vi "Lockin_Vsg.vi"(8 "error in (no error)":errorcluster, 11 "Transport":refnum<class "Transport.lvclass">) -> (0 "error out":errorcluster, 3 "Transport out":refnum<class "Transport.lvclass">)   [LabVIEW 2016, in "Transport.lvclass"]
uses:
  Transport.lvclass
  Control Experiment/Typedefs/Instruments--cluster.ctl
  <userlib>/LevyLab/Krohn Hite 7008/Instrument.KH7008.lvclass
  <userlib>/LevyLab/Lockin-Multichannel/Instrument.Lockin/Instrument.Lockin.lvclass
  <userlib>/LevyLab/Levylab Instruments/Instrument Types/Cryostat/Instrument.Cryostat.lvclass
  Transport.lvclass/Transport.ctl
  Control Experiment/Control Experiment.lvclass/Control Experiment.ctl
  subVI/LockinVsg Configuration--Cluster.ctl
  Control Experiment/Control Experiment.lvclass
panel:
  in  "Tab Control":enum32{"lockin/SG Control", "Data", "Other"}(tab)
  out "elapsed time (s)":u32=76
  in  "Side Gate Channel(s)":i32[](array[numeric])=[1]
  in  "Vmax (end)":dbl=0.1 format="%#_3p"
  in  "Vmin (start)":dbl format="%#_3p"
  in  "dV":dbl=0.001 format="%#_3p"
  in  "Experiment Comments":string="describe only the experiment you're doing right now"
  in  "Experiment Folder":string="Experiment folder"
  out "T (mK)":dbl
  in  "wait after setting Vsg (ms)":u32
  in  "Initial wait (ms)":u32=1000
  in  "Physical Channel":tag="Dev2/ao0" caption="Back Gate Channel"
  in  "Sweep":enum16{"Vsg", "Vbg"}(ring)
  in  "cycles (1,2,...)":i32=1 min=1 step=1
  in  "phase":dbl
  out "Field (T)":dbl=0.5 format="%#_13g"
  in  "function (ramp)":enum16{"Ramp", "Triangle", "Sine"}(ring)
  in  "set \"Vsg\" to initial value?":bool
  out "time b/w points (ms)":u32=76
  in  "stop":bool
  out "X Lockins":cluster{dbl[], dbl[]}[](graph)
  out "X Lockins 2":cluster{dbl[], dbl[]}[](graph)
  out "G4T":cluster{dbl[], dbl[]}[](graph)
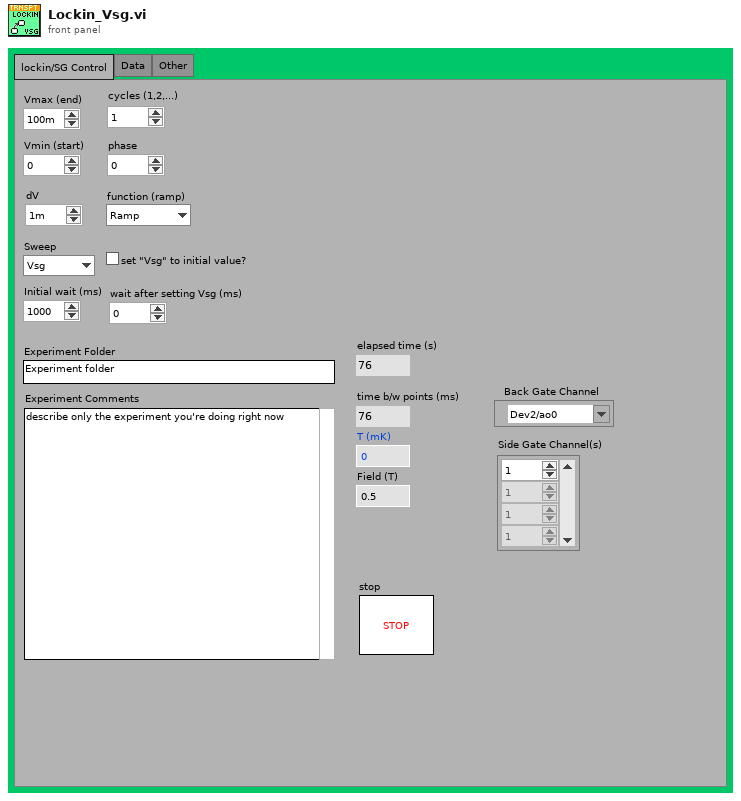
[diagram p1: front panel]
types:
  T1 = enum32{"Invalid", "Standard", "Closed", "Hidden", "Minimized", "Maximized"}
  T2 = enum32{"invalid app kind", "Development System", "Run Time System", "Student Edition", "Embedded LabVIEW", "Evaluation", "Custom"}
  T3 = typedef "Control Experiment.lvclass/Instruments--cluster.ctl" = cluster{"KH7008":refnum<class "Instrument.KH7008.lvclass">, "Lockin":refnum<class "Instrument.Lockin.lvclass">, "Temperature":refnum<class "Instrument.Cryostat.lvclass">, "Magnet":refnum<class "Instrument.Cryostat.lvclass">, "Rotator":refnum<class "Instrument.Cryostat.lvclass">, "Level":refnum<class "Instrument.Cryostat.lvclass">}
  T4 = cluster{"Core":cluster{"Current VI Reference":refnum<vi>, "Close Panel on Exit?":bool}, "Transport":refnum<class "Transport.lvclass">, "SweepControl":refnum<class "SweepControl.lvclass">, "Control Experiment":refnum<class "Control Experiment.lvclass">, "Instruments":T3, "Time":dbl, "Temperature":dbl, "Magnet":dbl, "Sweep Values":dbl[], "Results":dbl[][], "X Results":dbl[], "Y Results":dbl[], "X Results (all)":dbl[][], "Y Results (all)":dbl[][], "size":i32, "index":i32, "ms [0]":u32, "ms [i]":u32}
  T5 = cluster{"Current VI Reference":refnum<vi>, "Close Panel on Exit?":bool}
  T6 = enum32{"Bad", "Idle", "Run top level", "Running"}
  T7 = cluster{"I-":i32, "I+":i32, "V1-":i32, "V1+":i32, "V2-":i32, "V2+":i32}
  T8 = typedef "Transport.lvclass/LockinVsg Configuration--Cluster.ctl" = cluster{"Vsg Values":dbl[]}
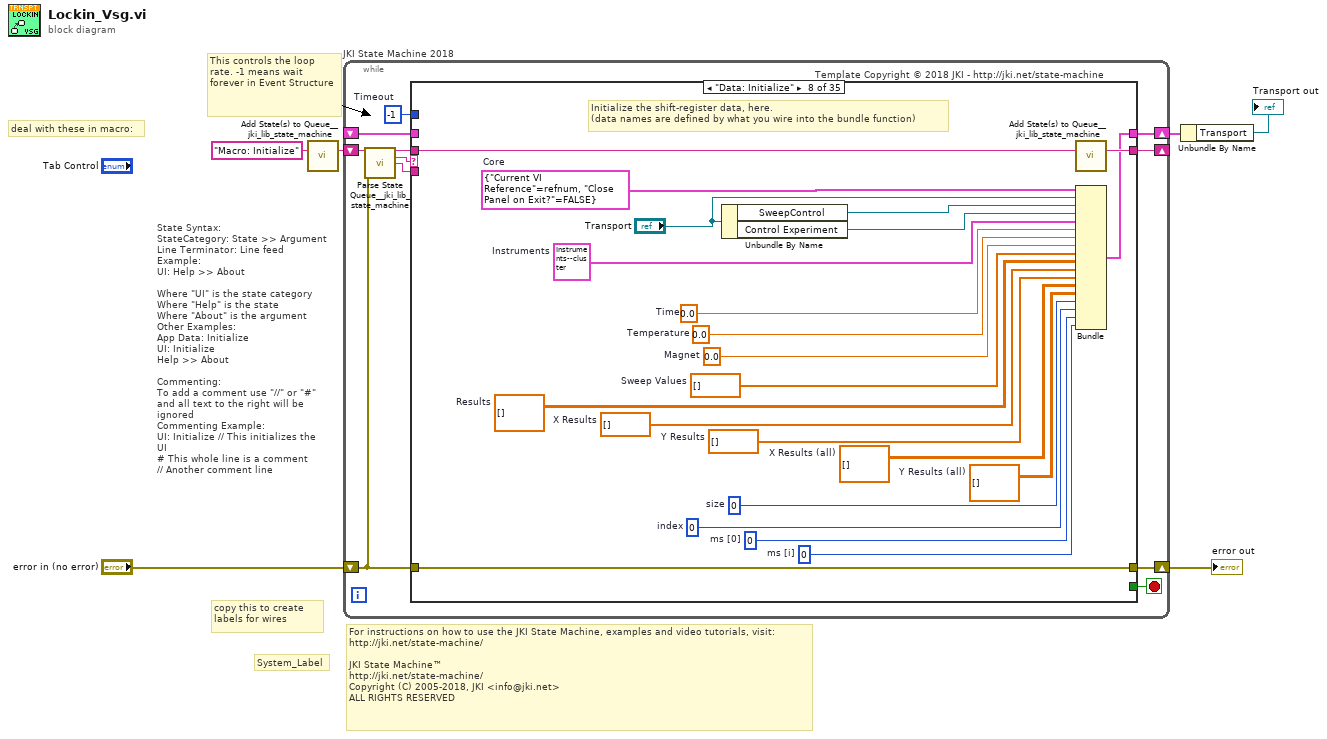
[diagram p0: block diagram]
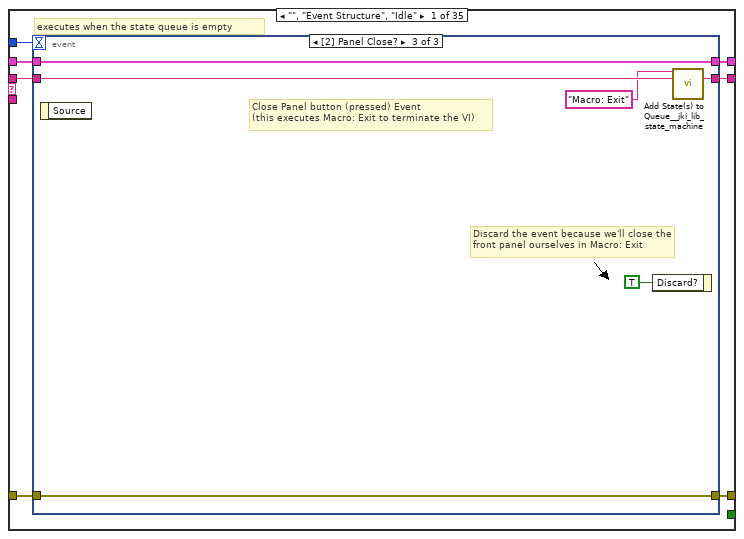
[diagram p2: hidden frame]
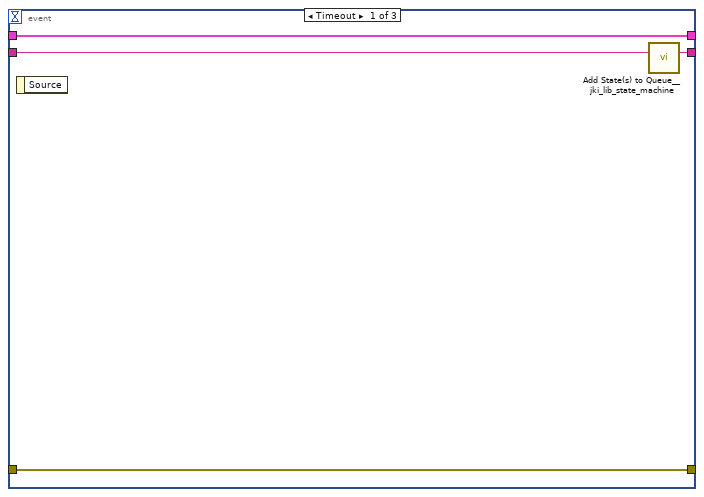
[diagram p3: hidden frame]
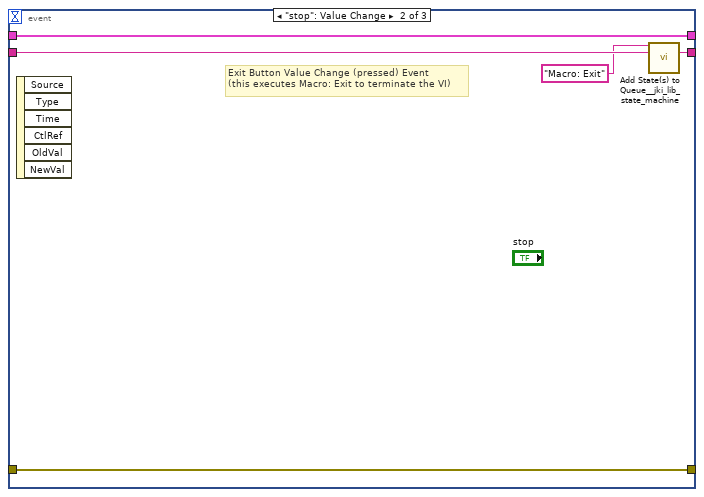
[diagram p4: hidden frame]
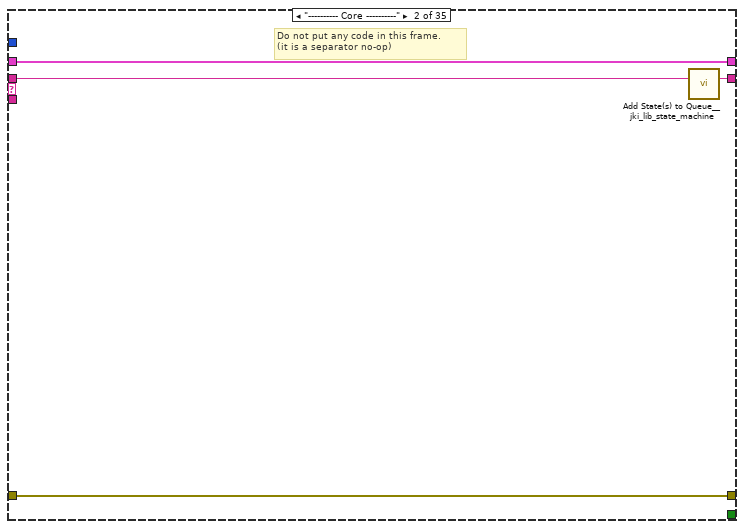
[diagram p5: hidden frame]
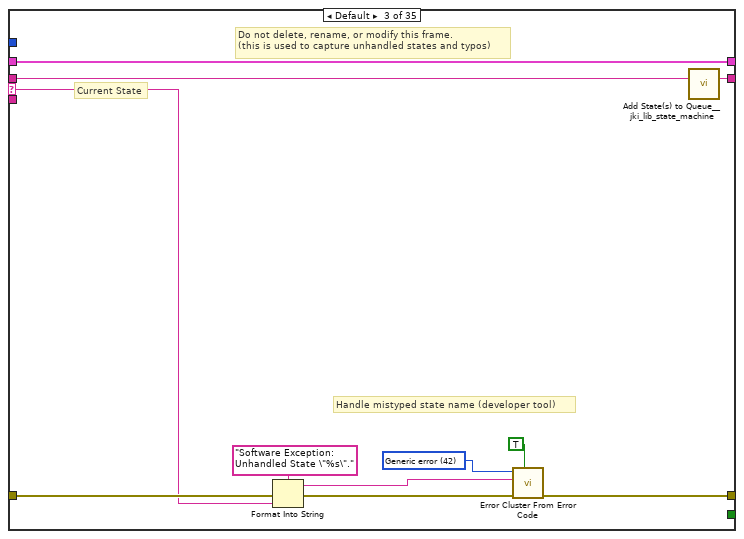
[diagram p6: hidden frame]
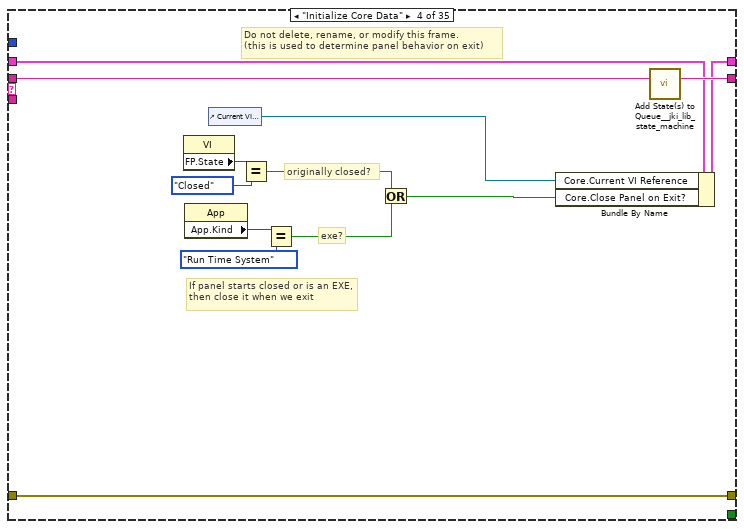
[diagram p7: hidden frame]
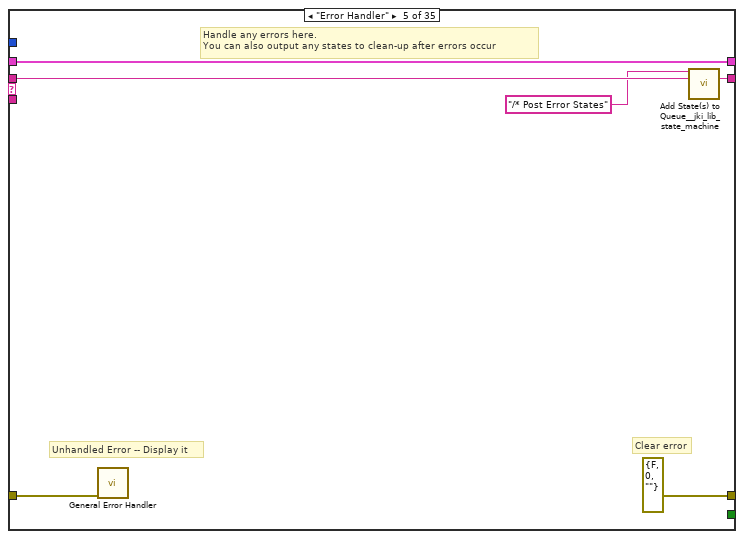
[diagram p8: hidden frame]
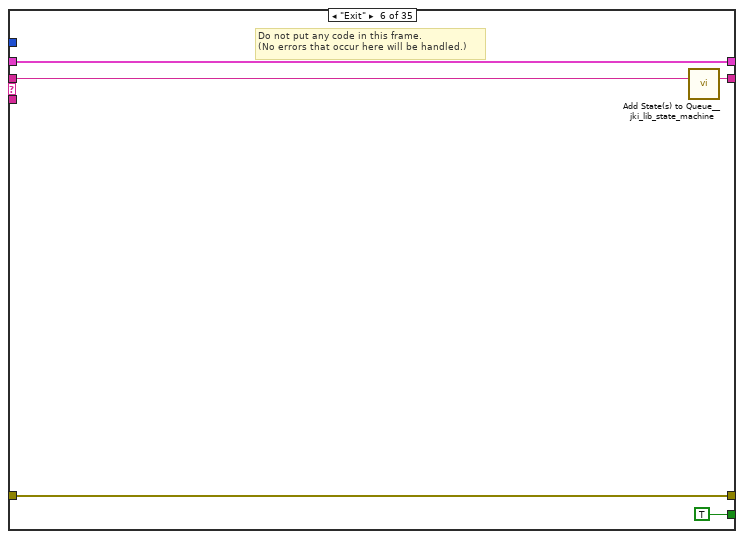
[diagram p9: hidden frame]
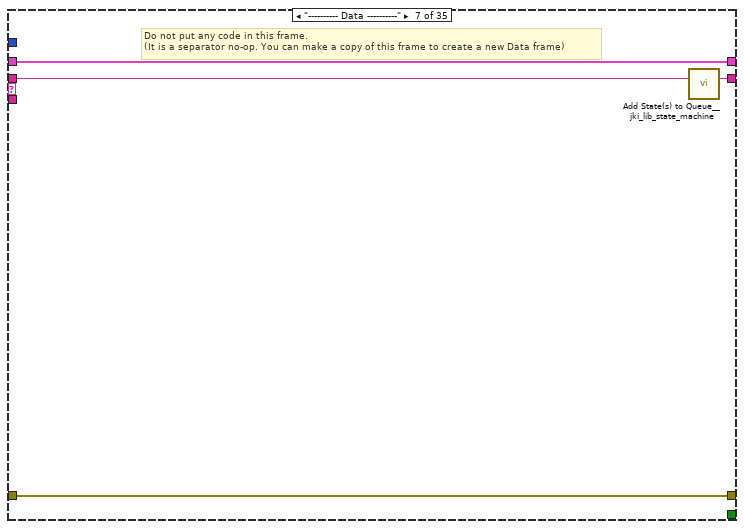
[diagram p10: hidden frame]
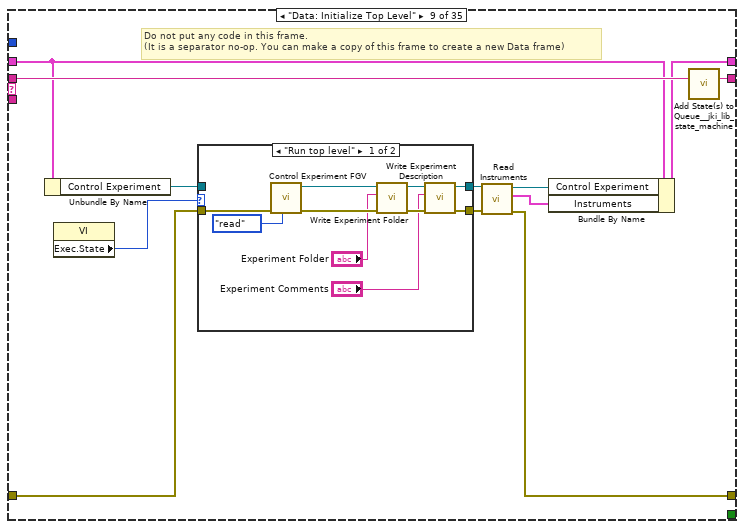
[diagram p11: hidden frame]
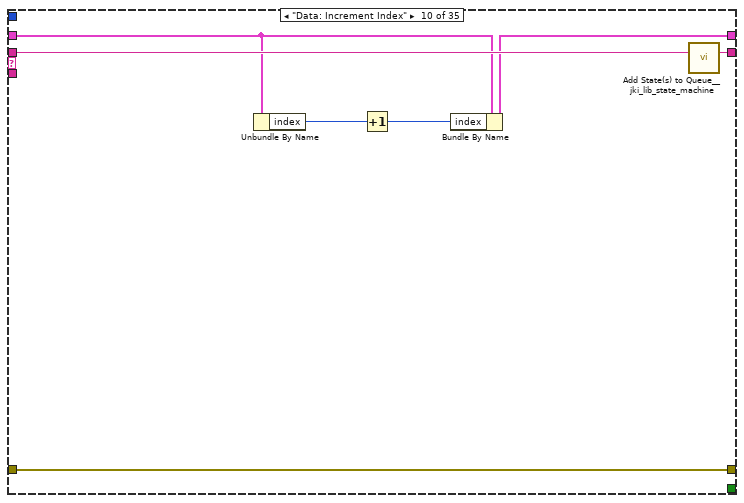
[diagram p13: hidden frame]
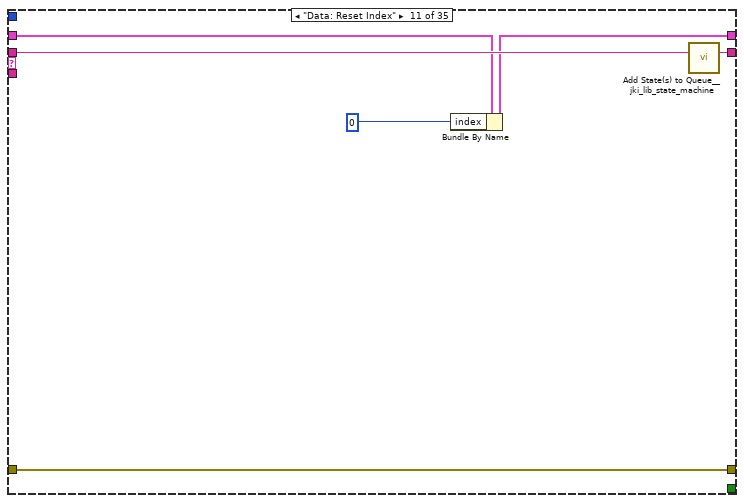
[diagram p14: hidden frame]
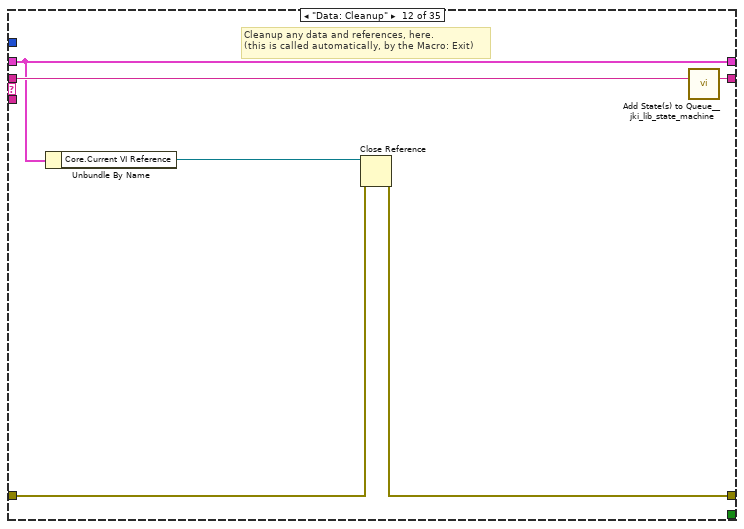
[diagram p15: hidden frame]
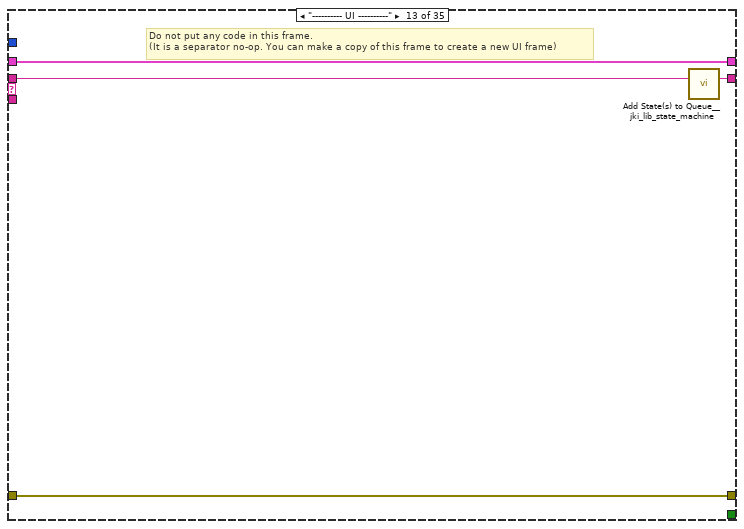
[diagram p16: hidden frame]
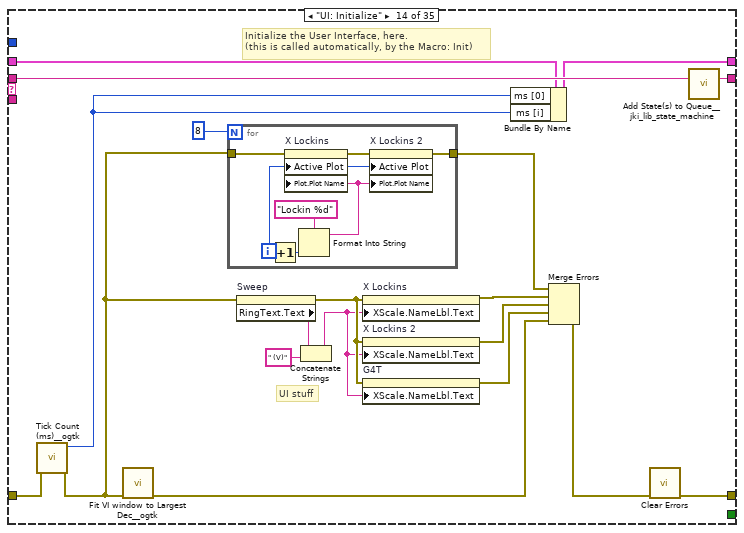
[diagram p17: hidden frame]
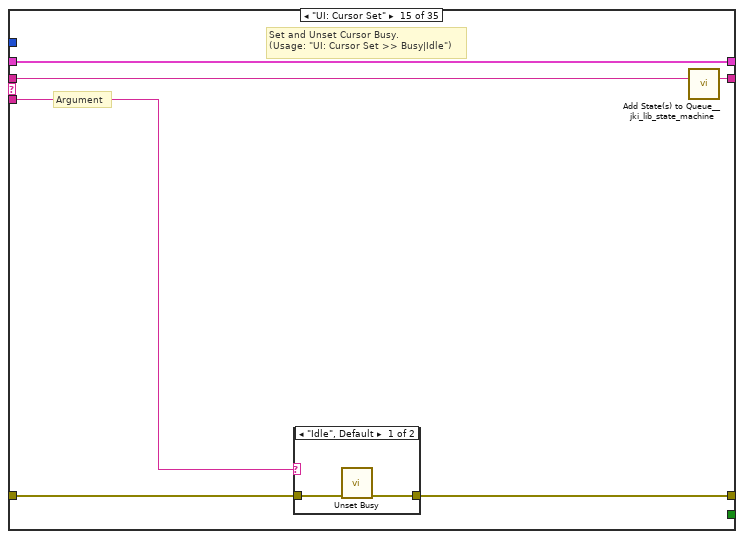
[diagram p18: hidden frame]
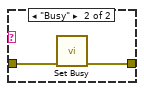
[diagram p19: hidden frame]
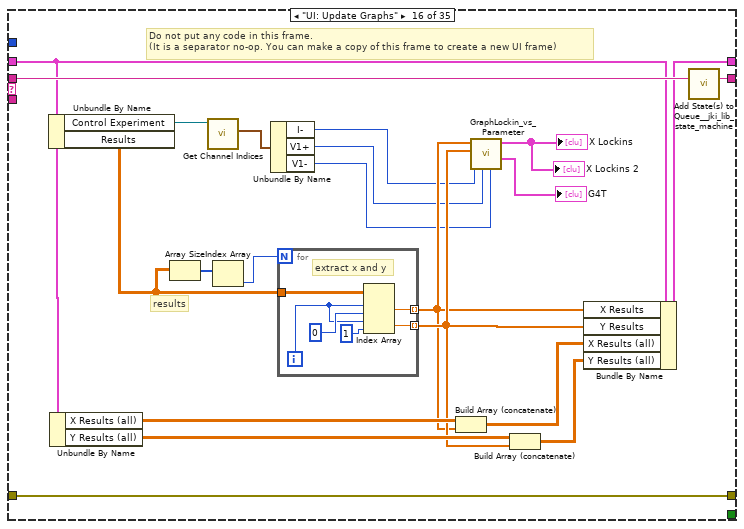
[diagram p20: hidden frame]
diagram:
  # "deal with these in macro:"
  # "For instructions on how to use the JKI State Machine, examples and video tutorials, visit:\nhttp://jki.net/state-machine/\n\nJKI State Machine™\nhttp://jki.net/state-machine/\nCopyright (C) 2005-2018, JKI <info@jki.net>\nALL RIGHTS RESERVED"
  # "State Syntax:\nStateCategory: State >> Argument\nLine Terminator: Line feed\nExample:\nUI: Help >> About\n\nWhere \"UI\" is the state category\nWhere \"Help\" is the state\nWhere \"About\" is the argument\nOther Examples:\nApp Data: Initialize\nUI: Initialize\nHelp >> About\n\nCommenting:\nTo add a comment use \"//\" or \"#\" and all text to the right will be ignored\nCommenting Example:\nUI: Initialize // This initializes the UI\n# This whole line is a comment\n// Another comment line"
  # "copy this to create labels for wires"
  # "This controls the loop rate. -1 means wait forever in Event Structure"
  # "System_Label"
  n1 = call <vilib>:"Add State(s) to Queue__jki_lib_state_machine.vi"("State(s) in (\"\")"="Macro: Initialize") -> ("States Out"=w6:string)  [unwired: 14 in]
  n2 = while "JKI State Machine 2018" {
    shift-right: [w10] -> w4
    shift-left: _ -> [w9]
    shift-right: [w13] -> w2
    shift-left: "error in (no error)" -> [w7]
    shift-right: [w12] -> _
    shift-left: w6 -> [w14]
    stop <- w11 stop-if-true
    w8 = -1  # Timeout
    # "Template Copyright © 2018 JKI - http://jki.net/state-machine"
    n3 = call <vilib>:"Parse State Queue__jki_lib_state_machine.vi"("State Queue"=w14, "Error In (no error)"=w7) -> ("Remaining States"=w16:string, "Current State"=w17:string, "Arguments"=w15:string)  [unwired: 11 in]
    n4 = case shown="\"Data: Initialize\"" w17 {
      selector: w17 -> [_ _ w44 _ _ _ _ _ _ _ _ _ _ _ _ _ _ _ _ _ _ _ _ _ _ _ _ _ _ _ _ _ _ _ _]
      tunnel: w16 -> [w24 w43 w48 w67 w73 w78 w82 w104 w116 w135 w141 w147 w151 w170 w183 w208 w227 w234 w303 w308 w326 w336 w340 w355 w359 w368 w378 w397 w408 w416 w423 w427 w431 w461 w480]
      tunnel: w15 -> [_ _ _ _ _ _ _ _ _ _ _ _ _ _ w178 _ _ w228 _ _ _ _ _ _ _ _ _ _ _ _ _ _ _ _ _]
      tunnel: w9 -> [w22 w40 w46 w60 w70 w76 w79 _ w106 w129 w138 w142 w148 w154 w181 w201 w222 w230 w300 w306 w318 w333 w337 w344 w356 w366 w376 w394 w401 w411 w419 w424 w428 w444 w476]
      tunnel: [w21 w41 w50 w64 errorcluster {"status"=FALSE, "code"=0, "source"=""} ("error out") w75 w80 w101 w107 w133 w139 w143 w149 w159 w179 w206 w215 w231 w301 w304 w324 w334 w338 w353 w357 w360 w373 w395 w402 w413 w421 w425 w429 w438 w474] -> w13
      tunnel: w7 -> [w20 w41 w49 w64 w69 w75 w80 w101 w108 w133 w139 w144 w149 w156 w180 w206 w224 w232 w301 w304 w324 w334 w338 w353 w357 w361 w374 w395 w404 w414 w421 w425 w429 w439 w475]
      tunnel: [w23 w42 w47 w66 w72 w77 w81 w103 w115 w134 w140 w146 w150 w169 w182 w207 w226 w233 w302 w307 w325 w335 w339 w354 w358 w367 w377 w396 w407 w415 w422 w426 w430 w460 w479] -> w12
      tunnel: [_ _ _ _ _ TRUE _ _ _ _ _ _ _ _ _ _ _ _ _ _ _ _ _ _ _ _ _ _ _ _ _ _ _ _ _] -> w11
      tunnel: [w19 w40 w46 w65 w70 w76 w79 w102 w105 w132 w137 w142 w148 w153 w181 w202 w221 w230 w300 w306 w318 w333 w337 w343 w356 w366 w376 w394 w400 w410 w418 w424 w428 w444 w476] -> w10
      tunnel: w8 -> [w18 _ _ _ _ _ _ _ _ _ _ _ _ _ _ _ _ _ _ _ _ _ _ _ _ _ _ _ _ _ _ _ _ _ _]
      frame "", "Event Structure", "Idle" {
        # "executes when the state queue is empty"
        n5 = event shown="[2] Panel Close?" {
          selector: _ -> [_ _ _]
          dyn-events: _ -> [_ _ _]
          timeout: w18 -> [_ _ _]
          tunnel: w24 -> [w28 w33 w39]
          tunnel: [w27 w32 w38] -> w23
          tunnel: w22 -> [w25 w30 w36]
          tunnel: [w26 w31 w37] -> w21
          tunnel: w20 -> [w26 w31 w37]
          tunnel: [w25 w30 w36] -> w19
          event Timeout {
            n6 = event-data() -> ()  [unwired: 1 in, 1 out]
            n7 = call <vilib>:"Add State(s) to Queue__jki_lib_state_machine.vi"("State(s) in (\"\")"=w28) -> ("States Out"=w27:string)  [unwired: 14 in]
          }
          event "stop": Value Change {
            # "Exit Button Value Change (pressed) Event\n(this executes Macro: Exit to terminate the VI)"
            n8 = event-data() -> ()  [unwired: 1 in, 6 out]
            n9 = call <vilib>:"Add State(s) to Queue__jki_lib_state_machine.vi"("State(s) in Front (\"\")"="Macro: Exit", "State(s) in (\"\")"=w33) -> ("States Out"=w32:string)  [unwired: 13 in]
          }
          event Panel Close? {
            # "Discard the event because we'll close the front panel ourselves in Macro: Exit"
            # "Close Panel button (pressed) Event\n(this executes Macro: Exit to terminate the VI)"
            n10 = event-data() -> ()  [unwired: 1 in, 1 out]
            n11 = event-data("Discard?"=TRUE) -> ()  [unwired: 1 in, 1 out]
            n12 = call <vilib>:"Add State(s) to Queue__jki_lib_state_machine.vi"("State(s) in Front (\"\")"="Macro: Exit", "State(s) in (\"\")"=w39) -> ("States Out"=w38:string)  [unwired: 13 in]
          }
        }
      }
      frame "---------- Core ----------" {
        # "Do not put any code in this frame.\n(it is a separator no-op)"
        n13 = call <vilib>:"Add State(s) to Queue__jki_lib_state_machine.vi"("State(s) in (\"\")"=w43) -> ("States Out"=w42:string)  [unwired: 14 in]
      }
      frame Default {
        w53 = 42 items=["No error", "Argument error", "Memory is full", "Out of zone", "End of file", "File already open", "Generic file I/O error", "File not found", "File permission error", "Disk is full", "Duplicate path", "Too many files open", "System feature not enabled", "Resource file not found", "Cannot add resource", "Resource not found", "Image not found", "Image memory error", "Pen does not exist", "Config type invalid", "Config token not found", "Config parse error", "Config memory error", "Bad external code format", "Bad external code offset", "External code not present", "Null window", "Destroy window error", "Null menu", "Print aborted", "Bad print record", "Print driver error", "Windows error during printing", "Memory error during printing", "Print dialog error", "Generic print error", "Invalid device refnum", "Device not found", "Device parameter error", "Device unit error", "Cannot open device", "Device call aborted", "Generic error", "Cancelled by user", "Object ID too low", "Object ID too high", "Object not in heap", "Unknown heap", "Unknown object (invalid DefProc)", "Unknown object (DefProc not in table)", "Message out of range", "Invalid (null) method", "Unknown message", "Manager call not supported", "Bad address", "Network operation in progress", "Network operation timed out", "Connection is busy", "Network attribute not supported", "Network error", "Address in use", "System out of memory", "Connection aborted", "Connection refused", "Not connected", "Already connected", "Connection closed", "Initialization error (interapplication manager)", "Bad occurrence", "Wait on unbound occurrence handler", "Occurrence queue overflow", "Datalog type conflict", "Unused", "Unrecognized type (interapplication manager)", "Memory corrupt", "Failed to make temporary DLL", "Old CIN version", "Drag socket not found", "Failed to load drop-object", "Failed to register OLE object", "Failed to release OLE object", "Format specifier type mismatch", "Unknown format specifier", "Too few format specifiers", "Too many format specifiers", "Scan failed", "Newer CIN version", "Error converting to variant", "Runtime menu error", "Password tampered", "Variant attribute not found", "Incompatible variant data type", "Event data is not available", "Event Store is not present", "Occurrence is not found", "Event Queue is not created", "Event info is not available", "Refnum passed is NULL", "Error retrieving Class GUID", "Error retrieving CoClass GUID", "Error retrieving TypeLib GUID.", "Bad built application magic bytes.", "Specific driver is different from the specific driver associated with the Logical Name.", "There is no session opened to the class driver.", "Max Error", "MAX - Error with config objects", "MAX - Error loading configuration", "MAX - Group not supported"]
        # "Current State"
        # "Do not delete, rename, or modify this frame.\n(this is used to capture unhandled states and typos)"
        # "Handle mistyped state name (developer tool)"
        n14 = Format Into String(format string="Software Exception: Unhandled State \"%s\"." ("message"), error in=w49, w44) -> (resulting string=w52:string, error out=w51:errorcluster)  [unwired: 1 in]
        n15 = call <vilib>:"Error Cluster From Error Code.vi"("show call chain? (False)"=TRUE, "error in (no error)"=w51, "error message (\"\")"=w52, "error code (0)"=w53) -> ("error out"=w50:errorcluster)  [unwired: 5 in]
        n16 = call <vilib>:"Add State(s) to Queue__jki_lib_state_machine.vi"("State(s) in (\"\")"=w48) -> ("States Out"=w47:string)  [unwired: 14 in]
      }
      frame "Initialize Core Data" {
        # "Do not delete, rename, or modify this frame.\n(this is used to determine panel behavior on exit)"
        # "originally closed?"
        # "exe?"
        # "If panel starts closed or is an EXE, then close it when we exit"
        n17 = property class="VI"() -> ("FP.State"=w57:T1)  [unwired: 2 in, 2 out]
        n18 = property class="App"() -> ("App.Kind"=w63:T2)  [unwired: 2 in, 2 out]
        n19 = control-ref of="Current VI Reference"() -> (w58:refnum<vi>)
        n20 = Equal?(x=w57, y=T1."Closed" ("Front Panel Window:State")) -> (x = y?=w55:bool)
        n21 = Equal?(x=w63, y=T2."Run Time System" ("Application:Kind")) -> (x = y?=w61:bool)
        n22 = Or(x=w55, y=w61) -> (x .or. y?=w59:bool)
        n23 = Bundle By Name(cluster=w60, "Core.Current VI Reference"=w58, "Core.Close Panel on Exit?"=w59) -> (w65:T4)
        n24 = call <vilib>:"Add State(s) to Queue__jki_lib_state_machine.vi"("State(s) in (\"\")"=w67) -> ("States Out"=w66:string)  [unwired: 14 in]
      }
      frame "Error Handler" {
        # "Unhandled Error -- Display it"
        # "Handle any errors here.\nYou can also output any states to clean-up after errors occur"
        # "Clear error"
        n25 = call <vilib>:"General Error Handler.vi"("error in (no error)"=w69) -> ()  [unwired: 10 in, 5 out]
        n26 = call <vilib>:"Add State(s) to Queue__jki_lib_state_machine.vi"("State(s) in Front (\"\")"="/* Post Error States", "State(s) in (\"\")"=w73) -> ("States Out"=w72:string)  [unwired: 13 in]
      }
      frame "Exit" {
        # "Do not put any code in this frame.\n(No errors that occur here will be handled.)"
        n27 = call <vilib>:"Add State(s) to Queue__jki_lib_state_machine.vi"("State(s) in (\"\")"=w78) -> ("States Out"=w77:string)  [unwired: 14 in]
      }
      frame "---------- Data ----------" {
        # "Do not put any code in this frame.\n(It is a separator no-op. You can make a copy of this frame to create a new Data frame)"
        n28 = call <vilib>:"Add State(s) to Queue__jki_lib_state_machine.vi"("State(s) in (\"\")"=w82) -> ("States Out"=w81:string)  [unwired: 14 in]
      }
      frame "Data: Initialize" {
        w85 = 0  # size
        w86 = u32 0  # ms [i]
        w87 = u32 0  # ms [0]
        w91 = 0  # index
        w92 = dbl[][] []  # Y Results (all)
        w93 = dbl[][] []  # X Results (all)
        w88 = dbl[] []  # Y Results
        w89 = dbl[] []  # X Results
        w94 = 0.0  # Time
        w95 = dbl[][] []  # Results
        w96 = dbl[] []  # Sweep Values
        w97 = 0.0  # Magnet
        w90 = 0.0  # Temperature
        w98 = T3 {"KH7008"=refnum, "Lockin"=refnum, "Temperature"=refnum, "Magnet"=refnum, "Rotator"=refnum, "Level"=refnum}  # Instruments
        w100 = T5 {"Current VI Reference"=refnum, "Close Panel on Exit?"=FALSE}  # Core
        # "Initialize the shift-register data, here.\n(data names are defined by what you wire into the bundle function)"
        n29 = Unbundle By Name("Transport") -> ("SweepControl"=w84:refnum<class "SweepControl.lvclass">, "Control Experiment"=w83:refnum<class "Control Experiment.lvclass">)
        n30 = call <vilib>:"Add State(s) to Queue__jki_lib_state_machine.vi"("State(s) in (\"\")"=w104) -> ("States Out"=w103:string)  [unwired: 14 in]
        n31 = Bundle("Core"=w100, "Transport"="Transport", "SweepControl"=w84, "Control Experiment"=w83, "Instruments"=w98, "Time"=w94, "Temperature"=w90, "Magnet"=w97, "Sweep Values"=w96, "Results"=w95, "X Results"=w89, "Y Results"=w88, "X Results (all)"=w93, "Y Results (all)"=w92, "size"=w85, "index"=w91, "ms [0]"=w87, "ms [i]"=w86) -> (w102:T4)  [unwired: 1 in]
      }
      frame "Data: Initialize Top Level" {
        # "Do not put any code in this frame.\n(It is a separator no-op. You can make a copy of this frame to create a new Data frame)"
        n32 = Unbundle By Name(w106) -> ("Control Experiment"=w109:refnum<class "Control Experiment.lvclass">)
        n33 = property class="VI"() -> ("Exec.State"=w114:T6)  [unwired: 2 in, 2 out]
        n34 = case shown="\"Run top level\"" w114 {
          tunnel: w108 -> [w126 w127]
          tunnel: [w121 w127] -> w110
          tunnel: [w120 w128] -> w111
          tunnel: w109 -> [_ w128]
          frame "Run top level" {
            n35 = call "Control Experiment FGV.vi"("Function"=enum16{"read", "write"}."read", "error in (no error)"=w126) -> ("error out"=w124:errorcluster, "Control Experiment.lvclass out"=w125:refnum<class "Control Experiment.lvclass">)  [unwired: 8 in]
            n36 = call "Write Experiment Folder.vi"("error in (no error)"=w124, "Experiment Folder"="Experiment Folder", "Control Experiment in"=w125) -> ("error out"=w122:errorcluster, "Control Experiment out"=w123:refnum<class "Control Experiment.lvclass">)  [unwired: 7 in]
            n37 = call "Write Experiment Description.vi"("error in (no error)"=w122, "Experiment Description"="Experiment Comments", "Control Experiment in"=w123) -> ("error out"=w121:errorcluster, "Control Experiment out"=w120:refnum<class "Control Experiment.lvclass">)  [unwired: 7 in]
          }
          frame "Running", Default {
          }
        }
        n38 = call "Read Instruments.vi"("error in (no error)"=w110, "Control Experiment in"=w111) -> ("error out"=w107:errorcluster, "Instruments"=w113:T3, "Control Experiment out"=w112:refnum<class "Control Experiment.lvclass">)  [unwired: 7 in]
        n39 = Bundle By Name(cluster=w106, "Control Experiment"=w112, "Instruments"=w113) -> (w105:T4)
        n40 = call <vilib>:"Add State(s) to Queue__jki_lib_state_machine.vi"("State(s) in (\"\")"=w116) -> ("States Out"=w115:string)  [unwired: 14 in]
      }
      frame "Data: Increment Index" {
        n41 = Unbundle By Name(w129) -> ("index"=w131:i32)
        n42 = Increment(x=w131) -> (x+1=w130:i32)
        n43 = Bundle By Name(cluster=w129, "index"=w130) -> (w132:T4)
        n44 = call <vilib>:"Add State(s) to Queue__jki_lib_state_machine.vi"("State(s) in (\"\")"=w135) -> ("States Out"=w134:string)  [unwired: 14 in]
      }
      frame "Data: Reset Index" {
        n45 = Bundle By Name(cluster=w138, "index"=0) -> (w137:T4)
        n46 = call <vilib>:"Add State(s) to Queue__jki_lib_state_machine.vi"("State(s) in (\"\")"=w141) -> ("States Out"=w140:string)  [unwired: 14 in]
      }
      frame "Data: Cleanup" {
        # "Cleanup any data and references, here.\n(this is called automatically, by the Macro: Exit)"
        n47 = Unbundle By Name(w142) -> ("Core.Current VI Reference"=w145:refnum<vi>)
        n48 = Close Reference(reference=w145, error in (no error)=w144) -> (error out=w143:errorcluster)
        n49 = call <vilib>:"Add State(s) to Queue__jki_lib_state_machine.vi"("State(s) in (\"\")"=w147) -> ("States Out"=w146:string)  [unwired: 14 in]
      }
      frame "---------- UI ----------" {
        # "Do not put any code in this frame.\n(It is a separator no-op. You can make a copy of this frame to create a new UI frame)"
        n50 = call <vilib>:"Add State(s) to Queue__jki_lib_state_machine.vi"("State(s) in (\"\")"=w151) -> ("States Out"=w150:string)  [unwired: 14 in]
      }
      frame "UI: Initialize" {
        # "UI stuff"
        # "Initialize the User Interface, here.\n(this is called automatically, by the Macro: Init)"
        n51 = call <userlib>:"Tick Count (ms)__ogtk.vi"("error in (no error)"=w156) -> ("error out"=w155:errorcluster, "millisecond timer value"=w152:u32)  [unwired: 9 in]
        n52 = call <userlib>:"Fit VI window to Largest Dec__ogtk.vi"("error in (no error)"=w155) -> ("error out"=w158:errorcluster)  [unwired: 5 in, 1 out]
        n53 = for {
          N: 8 -> [_]
          tunnel: [w171] -> w165
          tunnel: w155 -> [w176]
          i -> [w174]
          n54 = Increment(x=w174) -> (x+1=w172:i32)
          n55 = Format Into String(format string="Lockin %d", w172) -> (resulting string=w175:string)  [unwired: 2 in, 1 out]
          n56 = property on="X Lockins" class="XYGraph (strict)"(error in=w176, "Active Plot"=w174, "Plot.Plot Name"=w175) -> (error out=w173:errorcluster)  [unwired: 1 in, 1 out]
          n57 = property on="X Lockins 2" class="XYGraph (strict)"(error in=w173, "Active Plot"=w174, "Plot.Plot Name"=w175) -> (error out=w171:errorcluster)  [unwired: 1 in, 1 out]
        }
        n58 = property on="Sweep" class="Enum (strict)"(error in=w155) -> (error out=w164:errorcluster, "RingText.Text"=w162:string)  [unwired: 1 in, 1 out]
        n59 = Concatenate Strings(w162, " (V)" ("string")) -> (w163:string)
        n60 = property on="X Lockins" class="XYGraph (strict)"(error in=w164, "XScale.NameLbl.Text"=w163) -> (error out=w166:errorcluster)  [unwired: 1 in, 1 out]
        n61 = property on="X Lockins 2" class="XYGraph (strict)"(error in=w164, "XScale.NameLbl.Text"=w163) -> (error out=w167:errorcluster)  [unwired: 1 in, 1 out]
        n62 = property on="G4T" class="XYGraph (strict)"(error in=w164, "XScale.NameLbl.Text"=w163) -> (error out=w168:errorcluster)  [unwired: 1 in, 1 out]
        n63 = Bundle By Name(cluster=w154, "ms [0]"=w152, "ms [i]"=w152) -> (w153:T4)
        n64 = Merge Errors(w165, w166, w167, w168, w158) -> (w157:errorcluster)
        n65 = call <vilib>:"Clear Errors.vi"("error in (no error)"=w157) -> ("error out"=w159:errorcluster)  [unwired: 5 in, 1 out]
        n66 = call <vilib>:"Add State(s) to Queue__jki_lib_state_machine.vi"("State(s) in (\"\")"=w170) -> ("States Out"=w169:string)  [unwired: 14 in]
      }
      frame "UI: Cursor Set" {
        # "Argument"
        # "Set and Unset Cursor Busy.\n(Usage: \"UI: Cursor Set >> Busy|Idle\")"
        n67 = case shown="\"Idle\", Default" w178 {
          tunnel: w180 -> [w185 w187]
          tunnel: [w184 w186] -> w179
          frame "Idle", Default {
            n68 = call <vilib>:"Unset Busy.vi"("error in (no error)"=w185) -> ("error out"=w184:errorcluster)  [unwired: 10 in]
          }
          frame "Busy" {
            n69 = call <vilib>:"Set Busy.vi"("error in (no error)"=w187) -> ("error out"=w186:errorcluster)  [unwired: 9 in, 1 out]
          }
        }
        n70 = call <vilib>:"Add State(s) to Queue__jki_lib_state_machine.vi"("State(s) in (\"\")"=w183) -> ("States Out"=w182:string)  [unwired: 14 in]
      }
      frame "UI: Update Graphs" {
        # "results"
        # "Do not put any code in this frame.\n(It is a separator no-op. You can make a copy of this frame to create a new UI frame)"
        n71 = Unbundle By Name(w201) -> ("Control Experiment"=w192:refnum<class "Control Experiment.lvclass">, "Results"=w197:dbl[][])
        n72 = Unbundle By Name(w201) -> ("X Results (all)"=w200:dbl[][], "Y Results (all)"=w196:dbl[][])
        n73 = Array Size(array=w197) -> (size(s)=w204:i32[])
        n74 = call "Get Channel Indices.vi"("Control Experiment in"=w192) -> ("Indices"=w191:T7)  [unwired: 8 in, 2 out]
        n75 = Index Array(array=w204) -> (element=w203:i32)  [unwired: 1 in]
        n76 = Unbundle By Name(w191) -> ("I-"=w188:i32, "V1+"=w190:i32, "V1-"=w189:i32)
        n77 = for {
          N: w203 -> [_]
          tunnel: w197 -> [w212]
          tunnel: [w211] -> w194 mode=indexing
          tunnel: [w210] -> w195 mode=indexing
          i -> [w209]
          # "extract x and y"
          n78 = Index Array(array=w212, index (row) #1=w209, index (col) #1=0 ("disabled index (col)"), index (row) #2=w209, index (col) #2=1 ("disabled index (col)")) -> (element #1=w211:dbl, element #2=w210:dbl)
        }
        n79 = Build Array (concatenate)(w200, w194) -> (w199:dbl[][])
        n80 = call "GraphLockin_vs_Parameter.vi"("V-"=w189, "V+"=w190, "Current"=w188, "Y[ ]"=w195, "X[ ]"=w194) -> ("G(e2/h) vs Parameter"=→"G4T":cluster{"Y":dbl[], "Y":dbl[]}[], "X vs Parameter"=→"X Lockins" →"X Lockins 2":cluster{dbl[], dbl[]}[])  [unwired: 3 in, 2 out]
        n81 = Build Array (concatenate)(w196, w195) -> (w198:dbl[][])
        n82 = Bundle By Name(cluster=w201, "X Results"=w194, "Y Results"=w195, "X Results (all)"=w199, "Y Results (all)"=w198) -> (w202:T4)
        n83 = call <vilib>:"Add State(s) to Queue__jki_lib_state_machine.vi"("State(s) in (\"\")"=w208) -> ("States Out"=w207:string)  [unwired: 14 in]
      }
      frame "UI: Update Timer" {
        n84 = Unbundle By Name(w222) -> ("ms [0]"=w223:u32)
        n85 = call <userlib>:"Tick Count (ms)__ogtk.vi"("error in (no error)"=w224) -> ("error out"=w216:errorcluster, "millisecond timer value"=w220:u32)  [unwired: 9 in]
        n86 = Subtract(x=w220, y=w223) -> (x-y=w218:u32)
        n87 = call <userlib>:"MGI Milliseconds Since Last Call.vi"("Error In"=w216) -> ("ms"=→"time b/w points (ms)":u32, "Error Out"=w215:errorcluster)  [unwired: 5 in]
        n88 = Multiply(x=w218, y=u32 1000 ("x")) -> (x*y=→"elapsed time (s)":u32)
        n89 = Bundle By Name(cluster=w222, "ms [i]"=w220) -> (w221:T4)
        n90 = call <vilib>:"Add State(s) to Queue__jki_lib_state_machine.vi"("State(s) in (\"\")"=w227) -> ("States Out"=w226:string)  [unwired: 14 in]
      }
      frame "UI: Front Panel State" {
        # "Argument"
        # "Set Front Panel Open or Closed\n(Usage: \"UI: Front Panel State >> Open|Close\")"
        n91 = Unbundle By Name(w230) -> ("Core.Current VI Reference"=w229:refnum<vi>)
        n92 = case shown="\"Minimize\", \"Minimized\"" w228 {
          tunnel: w232 -> [w240 w255 w266 w279 w292]
          tunnel: [w242 w256 w268 w281 w294] -> w231
          tunnel: w229 -> [w241 w253 w267 w280 w293]
          frame "Open", "Standard", Default {
            w235 = T1."Standard" ("State")
            n93 = property class="VI"(reference=w241, error in=w240) -> (reference out=w238:refnum<vi>, error out=w239:errorcluster, "FP.State"=w237:T1)
            n94 = Not Equal?(x=w237, y=w235) -> (x != y?=w236:bool)
            n95 = case shown="True" w236 {
              tunnel: [w246 w248] -> w242
              tunnel: w239 -> [w245 w248]
              tunnel: w238 -> [w244 _]
              tunnel: w235 -> [w243 _]
              frame True {
                n96 = invoke class="VI" method="FP.Open"(reference=w244, error in=w245, "Activate"=TRUE, "State"=w243) -> (error out=w246:errorcluster)  [unwired: 1 in, 4 out]
              }
              frame False {
              }
            }
          }
          frame "Close", "Closed" {
            n97 = property class="VI"(reference=w253, error in=w255) -> (reference out=w252:refnum<vi>, error out=w254:errorcluster, "FP.State"=w250:T1)
            n98 = Not Equal?(x=w250, y=T1."Closed" ("Front Panel Window:State")) -> (x != y?=w249:bool)
            n99 = case shown="True" w249 {
              tunnel: [w257 w260] -> w256
              tunnel: w254 -> [w257 w259]
              tunnel: w252 -> [_ w258]
              frame False {
              }
              frame True {
                n100 = invoke class="VI" method="FP.Close"(reference=w258, error in=w259) -> (error out=w260:errorcluster)  [unwired: 1 in, 2 out]
              }
            }
          }
          frame "Hidden", "Hide" {
            w261 = T1."Hidden" ("State")
            n101 = property class="VI"(reference=w267, error in=w266) -> (reference out=w264:refnum<vi>, error out=w265:errorcluster, "FP.State"=w263:T1)
            n102 = Not Equal?(x=w263, y=w261) -> (x != y?=w262:bool)
            n103 = case shown="True" w262 {
              tunnel: [w272 w273] -> w268
              tunnel: w265 -> [w271 w273]
              tunnel: w264 -> [w270 _]
              tunnel: w261 -> [w269 _]
              frame True {
                n104 = invoke class="VI" method="FP.Open"(reference=w270, error in=w271, "State"=w269) -> (error out=w272:errorcluster)  [unwired: 2 in, 4 out]
              }
              frame False {
              }
            }
          }
          frame "Minimize", "Minimized" {
            w274 = T1."Minimized" ("State")
            n105 = property class="VI"(reference=w280, error in=w279) -> (reference out=w277:refnum<vi>, error out=w278:errorcluster, "FP.State"=w276:T1)
            n106 = Not Equal?(x=w276, y=w274) -> (x != y?=w275:bool)
            n107 = case shown="True" w275 {
              tunnel: [w285 w286] -> w281
              tunnel: w278 -> [w284 w286]
              tunnel: w277 -> [w283 _]
              tunnel: w274 -> [w282 _]
              frame True {
                n108 = invoke class="VI" method="FP.Open"(reference=w283, error in=w284, "State"=w282) -> (error out=w285:errorcluster)  [unwired: 2 in, 4 out]
              }
              frame False {
              }
            }
          }
          frame "Maximize", "Maximized" {
            w287 = T1."Maximized" ("State")
            n109 = property class="VI"(reference=w293, error in=w292) -> (reference out=w290:refnum<vi>, error out=w291:errorcluster, "FP.State"=w289:T1)
            n110 = Not Equal?(x=w289, y=w287) -> (x != y?=w288:bool)
            n111 = case shown="True" w288 {
              tunnel: [w298 w299] -> w294
              tunnel: w291 -> [w297 w299]
              tunnel: w290 -> [w296 _]
              tunnel: w287 -> [w295 _]
              frame True {
                n112 = invoke class="VI" method="FP.Open"(reference=w296, error in=w297, "State"=w295) -> (error out=w298:errorcluster)  [unwired: 2 in, 4 out]
              }
              frame False {
              }
            }
          }
        }
        n113 = call <vilib>:"Add State(s) to Queue__jki_lib_state_machine.vi"("State(s) in (\"\")"=w234) -> ("States Out"=w233:string)  [unwired: 14 in]
      }
      frame "---------- Macro ----------" {
        # "Do not put any code in this frame.\n(It is a separator no-op. You can make a copy of this frame to create a new Macro frame)"
        n114 = call <vilib>:"Add State(s) to Queue__jki_lib_state_machine.vi"("State(s) in (\"\")"=w303) -> ("States Out"=w302:string)  [unwired: 14 in]
      }
      frame "Macro: Initialize" {
        # "Initialization Macro\n(This is called once, when the VI starts)"
        n115 = call <vilib>:"Add State(s) to Queue__jki_lib_state_machine.vi"("State(s) in Front (\"\")"="Data: Initialize\nInitialize Core Data\nUI: Initialize\nUI: Front Panel State >> Open\nData: Initialize Top Level\nData: Reset Index\nSweep: Initialize\nMacro: Sweep", "State(s) in (\"\")"=w308) -> ("States Out"=w307:string)  [unwired: 13 in]
      }
      frame "Macro: Sweep" {
        # "Do not put any code in this frame.\n(It is a separator no-op. You can make a copy of this frame to create a new Macro frame)"
        n116 = Unbundle By Name(w318) -> ("size"=w319:i32, "index"=w323:i32)
        n117 = Decrement(x=w319) -> (x-1=w311:i32)
        n118 = Not Equal?(x=w311, y=w323) -> (x != y?=w322:bool)
        n119 = Select(t="Data: Reset Index\nConfigure: Set" ("State(s) in Front (\"\")"), s="set \"Vsg\" to initial value?", f="" ("State(s) in Front (\"\")")) -> (s? t:f=w314:string)
        n120 = call <vilib>:"Add State(s) to Queue__jki_lib_state_machine.vi"("State(s) in Front (\"\")"="File: Save\nMacro: Exit" ("State(s) in Front (\"\")"), "State(s) at Back (\"\")"=w314) -> ("States Out"=w312:string)  [unwired: 13 in]
        n121 = Select(t="Macro: Sweep" ("State(s) in Front (\"\")"), s=w322, f=w312) -> (s? t:f=w321:string)
        n122 = call <vilib>:"Add State(s) to Queue__jki_lib_state_machine.vi"("State(s) in Front (\"\")"="Configure: Set\nConfigure: Wait\nMeasure: Lockin\nMeasure: Time\nMeasure: Cryostat\nUI: Update Graphs\nUI: Update Timer\nData: Increment Index" ("State(s) in Front (\"\")"), "State(s) at Back (\"\")"=w321) -> ("States Out"=w310:string)  [unwired: 13 in]
        n123 = call <vilib>:"Add State(s) to Queue__jki_lib_state_machine.vi"("State(s) in (\"\")"=w326, "State(s) at Back (\"\")"=w310) -> ("States Out"=w325:string)  [unwired: 13 in]
      }
      frame "Macro: Exit" {
        # "Exit Macro\n(This is called once, when the VI exits)"
        n124 = Unbundle By Name(w333) -> ("Core.Close Panel on Exit?"=w332:bool)
        n125 = Select(t="UI: Front Panel State >> Close", s=w332, f="") -> (s? t:f=w329:string)
        n126 = call <vilib>:"Add State(s) to Queue__jki_lib_state_machine.vi"("State(s) in (\"\")"=w329, "State(s) at Back (\"\")"="Data: Cleanup\nExit") -> ("States Out"=w327:string)  [unwired: 13 in]
        n127 = call <vilib>:"Add State(s) to Queue__jki_lib_state_machine.vi"("State(s) in Front (\"\")"=w327, "State(s) in (\"\")"=w336) -> ("States Out"=w335:string)  [unwired: 13 in]
      }
      frame "---------- Sweep ----------" {
        # "Do not put any code in this frame.\n(It is a separator no-op. You can make a copy of this frame to create a new Macro frame)"
        n128 = call <vilib>:"Add State(s) to Queue__jki_lib_state_machine.vi"("State(s) in (\"\")"=w340) -> ("States Out"=w339:string)  [unwired: 14 in]
      }
      frame "Sweep: Initialize" {
        # "define sweep"
        # "Do not put any code in this frame.\n(It is a separator no-op. You can make a copy of this frame to create a new Macro frame)"
        n129 = call <userlib>:"Max_Min_conversion.vi"("Min"="Vmin (start)", "Max"="Vmax (end)") -> ("offset"=w346:dbl, "Amplitude"=w345:dbl)  [unwired: 8 in]
        n130 = call <userlib>:"Ramp.vi"("phase"="phase", "function (ramp)"="function (ramp)", "cycles (1,2,...)"="cycles (1,2,...)", "step size"="dV", "offset"=w346, "amplitude"=w345) -> ("Waveform Graph"=w342:dbl[])  [unwired: 3 in, 2 out]
        n131 = Array Size(array=w342) -> (size(s)=w341:i32)
        n132 = Bundle By Name(cluster=w344, "Sweep Values"=w342, "size"=w341) -> (w343:T4)
        n133 = call <vilib>:"Add State(s) to Queue__jki_lib_state_machine.vi"("State(s) in (\"\")"=w355) -> ("States Out"=w354:string)  [unwired: 14 in]
      }
      frame "---------- Configure ----------" {
        # "Do not put any code in this frame.\n(It is a separator no-op. You can make a copy of this frame to create a new Macro frame)"
        n134 = call <vilib>:"Add State(s) to Queue__jki_lib_state_machine.vi"("State(s) in (\"\")"=w359) -> ("States Out"=w358:string)  [unwired: 14 in]
      }
      frame "Configure: Wait" {
        # "Do not put any code in this frame.\n(It is a separator no-op. You can make a copy of this frame to create a new Macro frame)"
        n135 = First Call?() -> (First Call?: T/F=w362:bool)
        n136 = Select(t="Initial wait (ms)", s=w362, f="wait after setting Vsg (ms)") -> (s? t:f=w365:u32)
        n137 = call <userlib>:"Wait (ms)__ogtk.vi"("error in (no error)"=w361, "milliseconds to wait"=w365) -> ("error out"=w360:errorcluster)  [unwired: 8 in, 1 out]
        n138 = call <vilib>:"Add State(s) to Queue__jki_lib_state_machine.vi"("State(s) in (\"\")"=w368) -> ("States Out"=w367:string)  [unwired: 14 in]
      }
      frame "Configure: Set" {
        # "Do not put any code in this frame.\n(It is a separator no-op. You can make a copy of this frame to create a new Macro frame)"
        n139 = Unbundle By Name(w376) -> ("Instruments.Lockin"=w375:refnum<class "Instrument.Lockin.lvclass">, "Sweep Values"=w372:dbl[], "index"=w371:i32)
        n140 = Index Array(array=w372, index=w371) -> (element=w370:dbl)
        n141 = case shown="\"Vsg\", Default" "Sweep" {
          tunnel: w375 -> [w383 _]
          tunnel: w374 -> [w381 w392]
          tunnel: [w380 w390] -> w373
          tunnel: w370 -> [w379 w391]
          frame "Vsg", Default {
            n142 = for {
              tunnel: "Side Gate Channel(s)" -> [w388] mode=indexing
              tunnel: w379 -> [w387]
              tunnel: w383 -> [w389]
              tunnel: [w384] -> _
              tunnel: w381 -> [w386]
              tunnel: [w385] -> w380
              n143 = call <userlib>:"configAO_DC.vi"("error in (no error)"=w386, "DC (V)"=w387, "AO Channel"=w388, "Instrument.Lockin in"=w389) -> ("error out"=w385:errorcluster, "Instrument.Lockin out"=w384:refnum<class "Instrument.Lockin.lvclass">)  [unwired: 6 in]
            }
          }
          frame "Vbg" {
            n144 = call <vilib>:"Voltage Update.vi"("error in (no error)"=w392, "Voltage Output"=w391, "Physical Channel"="Physical Channel") -> ("error out"=w390:errorcluster)  [unwired: 7 in, 1 out]
          }
        }
        n145 = call <vilib>:"Add State(s) to Queue__jki_lib_state_machine.vi"("State(s) in (\"\")"=w378) -> ("States Out"=w377:string)  [unwired: 14 in]
      }
      frame "---------- Measure ----------" {
        # "Template Separator\n(You can make a copy of, or modify, this frame)"
        n146 = call <vilib>:"Add State(s) to Queue__jki_lib_state_machine.vi"("State(s) in (\"\")"=w397) -> ("States Out"=w396:string)  [unwired: 14 in]
      }
      frame "Measure: Cryostat" {
        # "Your code here.\n(You can make a copy of, or modify, this frame)"
        n147 = Unbundle By Name(w401) -> ("Instruments.Magnet"=w405:refnum<class "Instrument.Cryostat.lvclass">, "Instruments.Temperature"=w406:refnum<class "Instrument.Cryostat.lvclass">)
        n148 = call-dynamic "Get Temperature.vi"("error in (no error)"=w404, "Instrument.Cryostat in"=w406) -> ("error out"=w403:errorcluster, "Temperature (K)"=w399:dbl)  [unwired: 6 in, 2 out]
        "T (mK)" <- w399
        n149 = call-dynamic "Get Magnet Field.vi"("error in (no error)"=w403, "Instrument.Cryostat in"=w405) -> ("error out"=w402:errorcluster, "B Field (T)"=w398:dbl)  [unwired: 6 in, 2 out]
        "Field (T)" <- w398
        n150 = Bundle By Name(cluster=w401, "Temperature"=w399, "Magnet"=w398) -> (w400:T4)
        n151 = call <vilib>:"Add State(s) to Queue__jki_lib_state_machine.vi"("State(s) in (\"\")"=w408) -> ("States Out"=w407:string)  [unwired: 14 in]
      }
      frame "Measure: Lockin" {
        # "Template Separator\n(You can make a copy of, or modify, this frame)"
        n152 = Unbundle By Name(w411) -> ("Instruments.Lockin"=w412:refnum<class "Instrument.Lockin.lvclass">)
        n153 = call <userlib>:"waitForNewResults.vi"("error in (no error)"=w414, "Instrument.Lockin in"=w412) -> ("error out"=w413:errorcluster, "Results"=w409:dbl[][])  [unwired: 7 in, 1 out]
        n154 = Bundle By Name(cluster=w411, "Results"=w409) -> (w410:T4)
        n155 = call <vilib>:"Add State(s) to Queue__jki_lib_state_machine.vi"("State(s) in (\"\")"=w416) -> ("States Out"=w415:string)  [unwired: 14 in]
      }
      frame "Measure: Time" {
        # "Your code here.\n(You can make a copy of, or modify, this frame)"
        n156 = Get Date/Time In Seconds() -> (seconds since 1Jan1904=w420:timestamp)
        n157 = To Double Precision Float(number=w420) -> (double precision float=w417:dbl)
        n158 = Bundle By Name(cluster=w419, "Time"=w417) -> (w418:T4)
        n159 = call <vilib>:"Add State(s) to Queue__jki_lib_state_machine.vi"("State(s) in (\"\")"=w423) -> ("States Out"=w422:string)  [unwired: 14 in]
      }
      frame "---------- File ----------" {
        # "Template Separator\n(You can make a copy of, or modify, this frame)"
        n160 = call <vilib>:"Add State(s) to Queue__jki_lib_state_machine.vi"("State(s) in (\"\")"=w427) -> ("States Out"=w426:string)  [unwired: 14 in]
      }
      frame "File: Configure" {
        # "Template Separator\n(You can make a copy of, or modify, this frame)"
        n161 = call <vilib>:"Add State(s) to Queue__jki_lib_state_machine.vi"("State(s) in (\"\")"=w431) -> ("States Out"=w430:string)  [unwired: 14 in]
      }
      frame "File: Save" {
        # "build cluster array"
        # "build cluster array(s) of multiple 1D data, dynamically name waves"
        # "build cluster array(s) of 1D data"
        # "build cluster array(s) of single values"
        # "Array:\nSweep"
        # "build data cluster array"
        # "build wavename array"
        # "Template Separator\n(You can make a copy of, or modify, this frame)"
        n162 = Unbundle By Name(w444) -> ("Sweep Values"=w435:dbl[])
        n163 = Unbundle By Name(w444) -> ("X Results (all)"=w446:dbl[][], "Y Results (all)"=w445:dbl[][])
        n164 = Unbundle By Name(w444) -> ("Control Experiment"=w432:refnum<class "Control Experiment.lvclass">, "Time"=w433:dbl, "Temperature"=w434:dbl, "Magnet"=w443:dbl)
        n165 = Transpose 2D Array(2D array=w446) -> (transposed array=w454:dbl[][])
        n166 = Transpose 2D Array(2D array=w445) -> (transposed array=w455:dbl[][])
        n167 = for {
          tunnel: w454 -> [w471] mode=indexing
          tunnel: w455 -> [w470] mode=indexing
          tunnel: [w469] -> w456 mode=concatenating
          tunnel: [w468] -> w457 mode=concatenating
          tunnel: [w466] -> w458 mode=indexing
          tunnel: [w463] -> w459 mode=indexing
          i -> [w467]
          n168 = Increment(x=w467) -> (x+1=w462:i32)
          n169 = Format Into String(format string="X%d" ("wavenames"), w462) -> (resulting string=w466:string)  [unwired: 2 in, 1 out]
          n170 = Build Cluster Array(w471) -> (w469:cluster{dbl[]}[])
          n171 = Build Cluster Array(w470) -> (w468:cluster{dbl[]}[])
          n172 = Format Into String(format string="Y%d" ("wavenames"), w462) -> (resulting string=w463:string)  [unwired: 2 in, 1 out]
        }
        n173 = Build Array(w443) -> (w440:dbl[])
        n174 = Build Array(w434) -> (w441:dbl[])
        n175 = Build Cluster Array(w435) -> (w451:cluster{"Sweep Values":dbl[]}[])
        n176 = Build Array("Vsg" ("wavenames")) -> (w450:string[])
        n177 = Build Array(w433) -> (w442:dbl[])
        n178 = Build Cluster Array(w442, w441, w440) -> (w447:cluster{dbl[]}[])
        n179 = Interleave 1D Arrays(w456, w457) -> (w449:cluster{dbl[]}[])
        n180 = Interleave 1D Arrays(w458, w459) -> (w448:string[])
        n181 = Build Array (concatenate)(w447, w451, w449) -> (w437:cluster{"Sweep Values":dbl[]}[])
        n182 = Build Array (concatenate)(string[] ["time", "T", "B"] ("wavenames (.Vx, etc)"), w450, w448) -> (w436:string[])
        n183 = call "Save Transport ITX File.vi"("error in (no error)"=w439, "Wavenames"=w436, "Data"=w437, "Control Experiment in"=w432) -> ("error out"=w438:errorcluster)  [unwired: 6 in, 1 out]
        n184 = call <vilib>:"Add State(s) to Queue__jki_lib_state_machine.vi"("State(s) in (\"\")"=w461) -> ("States Out"=w460:string)  [unwired: 14 in]
      }
      frame "File: JSON" {
        w477 = T8 {"Vsg Values"=[]}  # LockinVsg Sweep
        # "Template Separator\n(You can make a copy of, or modify, this frame)"
        n185 = Unbundle By Name(w476) -> ("Control Experiment"=w473:refnum<class "Control Experiment.lvclass">, "Sweep Values"=w472:dbl[])
        n186 = Bundle By Name(cluster=w477, "Vsg Values"=w472) -> (w478:T8)
        n187 = call "Save JSON File.vi"("error in (no error)"=w475, "Data"=w478, "Control Experiment in"=w473) -> ("error out"=w474:errorcluster)  [unwired: 8 in]
        n188 = call <vilib>:"Add State(s) to Queue__jki_lib_state_machine.vi"("State(s) in (\"\")"=w480) -> ("States Out"=w479:string)  [unwired: 14 in]
      }
    }
  }
  "error out" <- w2
  n189 = Unbundle By Name(w4) -> ("Transport"=→"Transport out":refnum<class "Transport.lvclass">)
